vi "Initialize Client.vi"(8 "error in (no error)":errorcluster, 11 "Client Controller in":refnum<class "Client Controller.lvclass">) -> (0 "error out":errorcluster, 3 "Client Controller out":refnum<class "Client Controller.lvclass">)   [LabVIEW 2016, in "Client Controller.lvlib" / "Client Controller.lvclass"]
uses:
  Client Controller.lvclass
  C:/Program Files (x86)/National Instruments/LabVIEW 2016/vi.lib/ActorFramework/Actor/Actor.lvclass
  <vilib>/ActorFramework/Actor/Actor.lvclass/Actor.ctl
  <vilib>/ActorFramework/Message Enqueuer/Message Enqueuer.lvclass/Message Enqueuer.ctl
  Client Controller.lvclass/Client Controller.ctl
  <vilib>/ActorFramework/Message Enqueuer/Enqueue.vi
  <vilib>/ActorFramework/Message Enqueuer/Init from Existing Queue.vi
  Messages/Negotiate Server Connection Msg/Negotiate Server Connection Msg.lvclass
  C:/Program Files (x86)/National Instruments/LabVIEW 2016/vi.lib/ActorFramework/Message/Message.lvclass
  <vilib>/ActorFramework/Stop Msg/Stop Msg.lvclass
  <vilib>/ActorFramework/Message Priority Queue/Priority Enqueue.vi
  <vilib>/ActorFramework/Message Enqueuer/Message Enqueuer.lvclass
  <vilib>/ActorFramework/Actor/Actor.lvclass
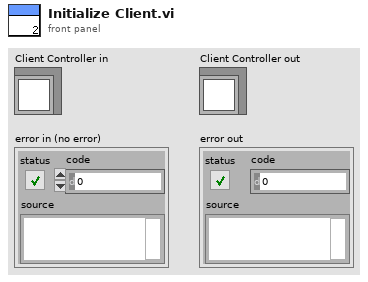
[diagram p1: front panel]
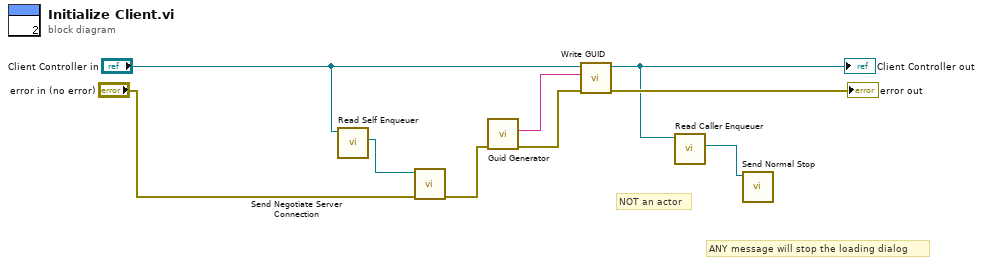
[diagram p0: block diagram]
diagram:
  # "NOT an actor"
  # "ANY message will stop the loading dialog"
  n1 = call <vilib>:"Read Self Enqueuer.vi"("Actor"="Client Controller in") -> ("Self Enqueuer"=w9:refnum<class "Message Enqueuer.lvclass">)  [unwired: 10 in]
  n2 = call "Send Negotiate Server Connection.vi"("error in (no error)"="error in (no error)", "Message Enqueuer"=w9) -> ("error out"=w6:errorcluster)  [unwired: 8 in, 1 out]
  n3 = call <vilib>:"Guid Generator.vi"("error in (no error)"=w6) -> ("error out"=w4:errorcluster, "GUID"=w5:string)  [unwired: 9 in]
  n4 = call "Write GUID.vi"("error in (no error)"=w4, "GUID"=w5, "Client Controller in"="Client Controller in") -> ("error out"=→"error out":errorcluster, "Client Controller out"=w2:refnum<class "Client Controller.lvclass">)  [unwired: 7 in]
  "Client Controller out" <- w2
  n5 = call <vilib>:"Read Caller Enqueuer.vi"("Actor"=w2) -> ("Caller Enqueuer"=w1:refnum<class "Message Enqueuer.lvclass">)  [unwired: 10 in]
  n6 = call <vilib>:"Send Normal Stop.vi"("Message Enqueuer"=w1) -> ()  [unwired: 10 in, 1 out]
